vi "Querey servo constants.vi"(8 "error in (no error)":errorcluster, 11 "connection in":variant) -> (0 "error out":errorcluster, 2 "Servo constants":T2={"Name"=enum."AxisX", "Pos position limit [mm]"=0.0, "Neg position limit [mm]"=0.0, "Pos velocity limit"=0.0, "Neg velocity limit"=0.0, "Acceleration limit"=0.0}, 3 "connection out":variant)   [LabVIEW 2017, in "Servo drive module.lvlib"]
doc: "Queries name, position and velocity limits."
uses:
  Servo drive module.lvlib
  ctl/Servo constants.ctl
  ctl/Axis names.ctl
  <vilib>/addons/eal4LabVIEW/eal4LabVIEW.lvlib
panel:
  in  "Aux Name":T1=enum."AxisX"
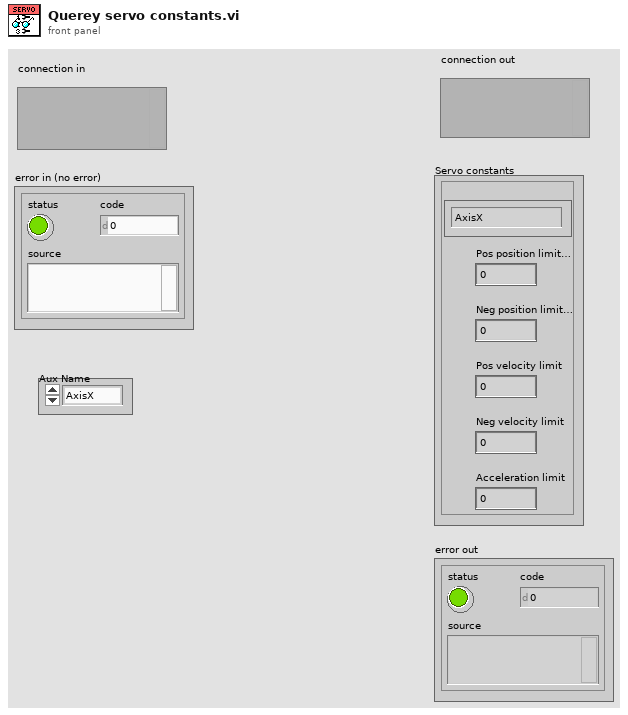
[diagram p1: front panel]
types:
  T1 = typedef "Servo drive module.lvlib/Axis names.ctl" = enum16{"Unknown", "AxisX", "AxisY", "AxisZ_left", "AxisZ_middle", "AxisZ_right"}
  T2 = typedef "Servo drive module.lvlib/Servo constants.ctl" = cluster{"Name":T1, "Pos position limit [mm]":dbl, "Neg position limit [mm]":dbl, "Pos velocity limit":dbl, "Neg velocity limit":dbl, "Acceleration limit":dbl}
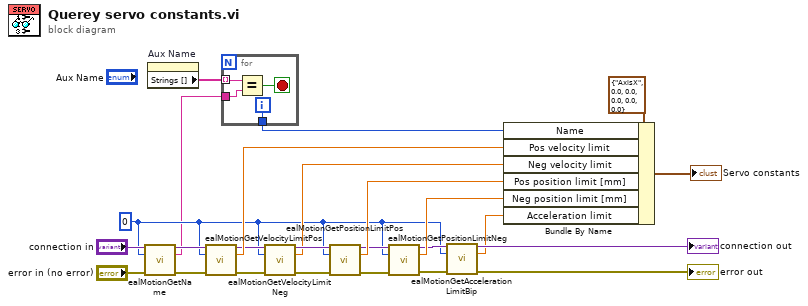
[diagram p0: block diagram]
diagram:
  w6 = 0 ("slave index")
  n1 = call <vilib>:"ealMotionGetName.vi"("connection in"="connection in", "slave index"=w6, "error in (no error)"="error in (no error)") -> ("connection out"=w13:variant, "name"=w1:string, "error out"=w19:errorcluster)  [unwired: 10 in]
  n2 = property on="Aux Name" class="Enum (strict)"() -> ("Strings []"=w2:string[])  [unwired: 2 in, 2 out]
  n3 = call <vilib>:"ealMotionGetVelocityLimitPos.vi"("connection in"=w13, "slave index"=w6, "error in (no error)"=w19) -> ("connection out"=w14:variant, "velocity limit pos."=w16:dbl, "error out"=w20:errorcluster)  [unwired: 10 in]
  n4 = for {
    tunnel: [w29] -> w3
    tunnel: w2 -> [w27] mode=indexing
    tunnel: w1 -> [w26]
    i -> [w29]
    stop <- w28 stop-if-true
    n5 = Equal?(x=w27, y=w26) -> (x = y?=w28:bool)
  }
  n6 = call <vilib>:"ealMotionGetVelocityLimitNeg.vi"("connection in"=w14, "slave index"=w6, "error in (no error)"=w20) -> ("connection out"=w22:variant, "negative velocity limit"=w17:dbl, "error out"=w21:errorcluster)  [unwired: 10 in]
  n7 = call <vilib>:"ealMotionGetPositionLimitPos.vi"("connection in"=w22, "slave index"=w6, "error in (no error)"=w21) -> ("connection out"=w10:variant, "positive position limit"=w23:dbl, "error out"=w12:errorcluster)  [unwired: 10 in]
  n8 = call <vilib>:"ealMotionGetPositionLimitNeg.vi"("connection in"=w10, "slave index"=w6, "error in (no error)"=w12) -> ("connection out"=w11:variant, "negative position limit"=w24:dbl, "error out"=w7:errorcluster)  [unwired: 10 in]
  n9 = call <vilib>:"ealMotionGetAccelerationLimitBip.vi"("connection in"=w11, "slave index"=w6, "error in (no error)"=w7) -> ("connection out"=→"connection out":variant, "bipolar acceration limit"=w4:dbl, "error out"=→"error out":errorcluster)  [unwired: 10 in]
  n10 = Bundle By Name(cluster=T2 {"Name"=enum."AxisX", "Pos position limit [mm]"=0.0, "Neg position limit [mm]"=0.0, "Pos velocity limit"=0.0, "Neg velocity limit"=0.0, "Acceleration limit"=0.0} ("Servo constants"), "Name"=w3, "Pos velocity limit"=w16, "Neg velocity limit"=w17, "Pos position limit [mm]"=w23, "Neg position limit [mm]"=w24, "Acceleration limit"=w4) -> (→"Servo constants":T2)
